vi "SRV_XModem_WriteFile_Comm.vi"(8 "error in (no error)":errorcluster, 10 "File Contents":string, 11 "SRV In":refnum<k5>) -> (0 "error out":errorcluster, 2 "reply to upload":string, 3 "SRV Out":refnum<k5>, 4 "## Reply":string, 6 "Replies":string[](array[string]))   [LabVIEW 2014]
doc: "Writes a file to the SRV.\n\n\nModified for Benilde St. Margaret's School - Tim Jump\nBy Doug Schmertman - Logic PD\nCopyright 2012"
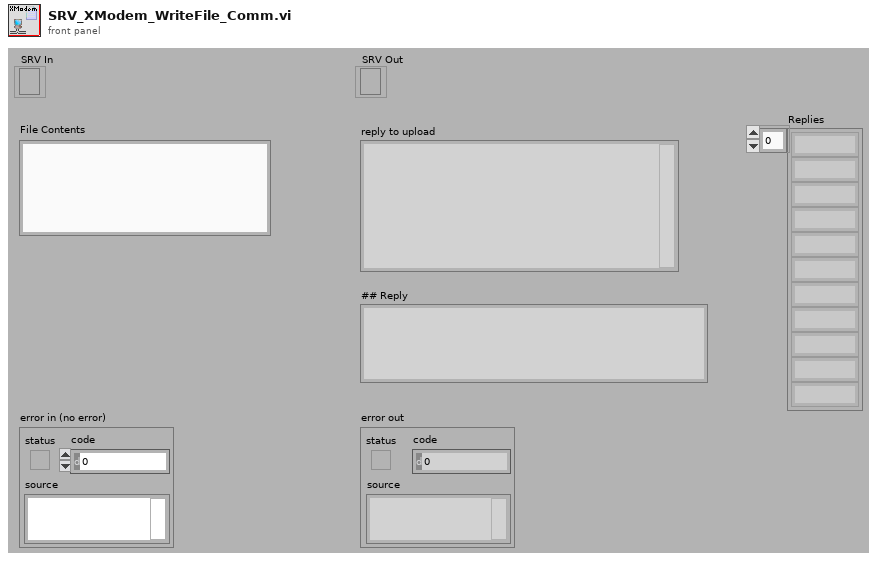
[diagram p1: front panel]
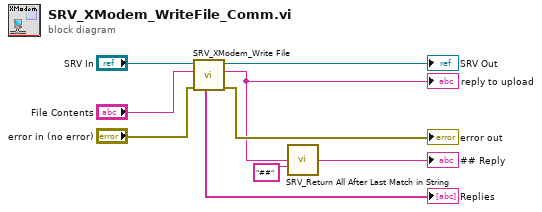
[diagram p0: block diagram]
diagram:
  n1 = call "SRV_XModem_Write File.vi"("error in"="error in (no error)", "file contents"="File Contents", "connection ID in"="SRV In") -> ("error out"=→"error out":errorcluster, "reply to upload"=w2:string, "connection ID"=→"SRV Out":refnum<k5>, "Replies"=→"Replies":string[])  [unwired: 4 in, 1 out]
  "reply to upload" <- w2
  n2 = call "SRV_Return All After Last Match in String.vi"("String"=w2, "String to Match"="##") -> ("Match Plus Remaining String"=→"## Reply":string)  [unwired: 13 in]
